vi "Test Oscillator A.vi"(8 "error in (no error)":errorcluster, 11 "VISA resource name":refnum<visa-resource-name>) -> (0 "error out":errorcluster, 3 "VISA resource name":refnum<visa-resource-name>)   [LabVIEW 2019, in "SR7270 Drivers.lvlib"]
uses:
  SR7270 Drivers.lvlib
  <userlib>/_OpenG.lib/numeric/numeric.llb/Random Number Within Range - DBL__ogtk.vi
  <vilib>/addons/_JKI Toolkits/Caraya/classes/Test/Test.lvclass
  <vilib>/addons/_JKI Toolkits/Caraya/classes/Assert/Assert.lvclass
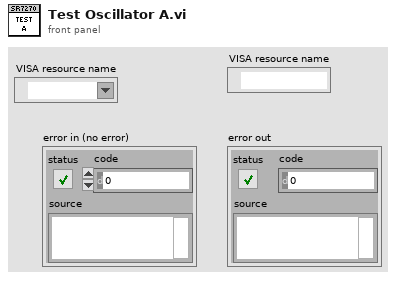
[diagram p1: front panel]
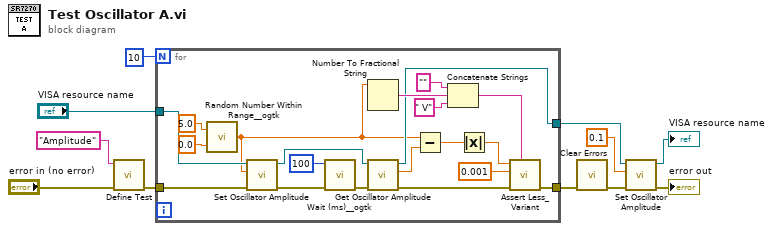
[diagram p0: block diagram]
diagram:
  n1 = call <vilib>:"Define Test.vi"("error in (no error)"="error in (no error)", "Label (VI Title)"="Amplitude") -> ("error out"=w7:errorcluster)  [unwired: 9 in]
  n2 = for {
    N: 10 -> [_]
    tunnel: "VISA resource name" -> [w17]
    tunnel: w7 -> [w23]
    tunnel: [w18] -> w11
    tunnel: [w15] -> w4
    n3 = call-poly <userlib>:"Random Number Within Range__ogtk.vi"("High"=5.0, "Low"=0.0) -> ("Random Number"=w14:dbl)  [unwired: 3 in]
    n4 = call "Set Oscillator Amplitude.vi"("error in (no error)"=w23, "Oscillator Amplitude (V)"=w14, "VISA resource name"=w17) -> ("error out"=w22:errorcluster, "VISA resource name out"=w16:refnum<visa-resource-name>)  [unwired: 7 in]
    n5 = call <userlib>:"Wait (ms)__ogtk.vi"("error in (no error)"=w22, "milliseconds to wait"=u32 100) -> ("error out"=w21:errorcluster)  [unwired: 8 in, 1 out]
    n6 = Number To Fractional String(number=w14) -> (F-format string=w28:string)  [unwired: 3 in]
    n7 = call "Get Oscillator Amplitude.vi"("error in (no error)"=w21, "VISA resource name"=w16) -> ("error out"=w20:errorcluster, "Oscillator Amplitude (V)"=w19:dbl, "VISA resource name out"=w15:refnum<visa-resource-name>)  [unwired: 7 in]
    n8 = Subtract(x=w14, y=w19) -> (x-y=w24:dbl)
    n9 = Concatenate Strings("" ("string"), w28, " V" ("string")) -> (w12:string)
    n10 = Absolute Value(x=w24) -> (abs(x)=w25:dbl)
    n11 = call <vilib>:"Assert Less_Variant.vi"("Label"=w12, "error in (no error)"=w20, "Y"=0.001 ("Phase (°)"), "X"=w25) -> ("error out"=w18:errorcluster)  [unwired: 7 in]
  }
  n12 = call <vilib>:"Clear Errors.vi"("error in (no error)"=w11) -> ("error out"=w6:errorcluster)  [unwired: 5 in, 1 out]
  n13 = call "Set Oscillator Amplitude.vi"("error in (no error)"=w6, "Oscillator Amplitude (V)"=0.1, "VISA resource name"=w4) -> ("error out"=→"error out":errorcluster, "VISA resource name out"=→"VISA resource name":refnum<visa-resource-name>)  [unwired: 7 in]
